vi "overlay enum on cell.vi"(4 "cell position":T1, 7 "Overlay?":bool, 8 "error in":errorcluster, 9 "Table Reference":refnum<vi>, 10 "current value":i32, 11 "Enum in":refnum<vi>) -> (0 "error out":errorcluster)   [LabVIEW 2013, in "Table Manager.lvlib"]
uses:
  Table Manager.lvlib
  <vilib>/Utility/miscctls.llb/LVRowAndColumnTypeDef.ctl
  <vilib>/Utility/miscctls.llb/LVPositionTypeDef.ctl
  Configuration Editor/Classes/EngineTags/EngineTags.lvclass
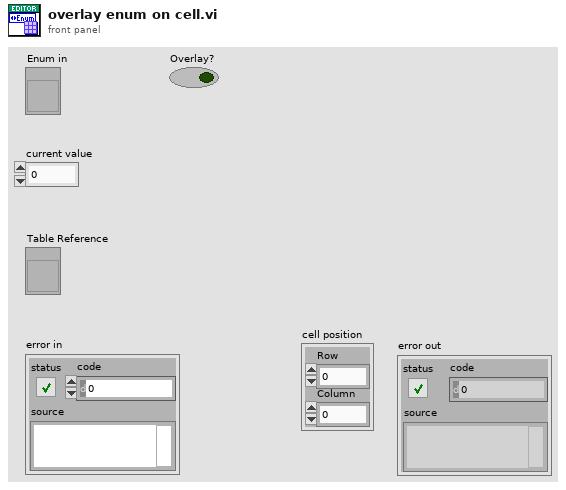
[diagram p1: front panel]
types:
  T1 = typedef "LVRowAndColumnTypeDef.ctl" = cluster{"Row":i32, "Column":i32}
  T2 = typedef "LVPositionTypeDef.ctl" = cluster{"Left":i32, "Top":i32}
  T3 = typedef "LVBoundsTypeDef.ctl" = cluster{"Width":u32, "Height":u32}
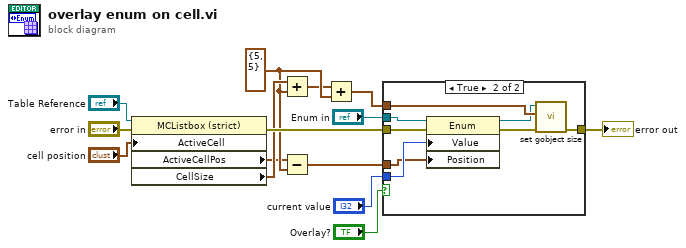
[diagram p0: block diagram]
diagram:
  w6 = T2 {"Left"=5, "Top"=5} ("Active Cell:Position")
  n1 = property class="MCListbox (strict)"(reference="Table Reference", error in="error in", "ActiveCell"="cell position") -> (error out=w12:errorcluster, "ActiveCellPos"=w5:T2, "CellSize"=w7:T3)  [unwired: 1 out]
  n2 = Add(x=w7, y=w6) -> (x+y=w3:T3)
  n3 = Subtract(x=w5, y=w6) -> (x-y=w13:T2)
  n4 = Add(x=w3, y=w6) -> (x+y=w4:T3)
  n5 = case shown="True" "Overlay?" {
    tunnel: w12 -> [w15 w19]
    tunnel: [w15 w23] -> w1
    tunnel: w4 -> [_ w22]
    tunnel: "current value" -> [_ w20]
    tunnel: w13 -> [_ w17]
    tunnel: "Enum in" -> [_ w16]
    frame False {
    }
    frame True {
      n6 = property on="Property Node" class="Enum"(reference=w16, error in=w19, "Value"=w20, "Position"=w17) -> (reference out=w21:refnum<vi>, error out=w18:errorcluster)
      n7 = call "set gobject size.vi"("error in"=w18, "size"=w22, "object refnum"=w21) -> ("error out"=w23:errorcluster)  [unwired: 8 in]
    }
  }
  "error out" <- w1
